vi "create_grid_from_corner_start.vi"(4 "y_step":dbl=0.1 format="%#_13g", 6 "x_step":dbl=0.1 format="%#_13g", 8 "y_n_pts":dbl=5.0 format="%#_13g", 9 "x_n_pts":dbl=5.0 format="%#_13g", 10 "y_start":dbl format="%#_13g", 11 "x_start":dbl format="%#_13g") -> (2 "Y":dbl[](array[numeric]), 3 "X":dbl[](array[numeric]))   [LabVIEW 2024]
uses:
  <vilib>/gmath/interp.llb/Create Mesh Grid (2D) (x,y arrays).vi
  <vilib>/gmath/NI_Gmath.lvlib
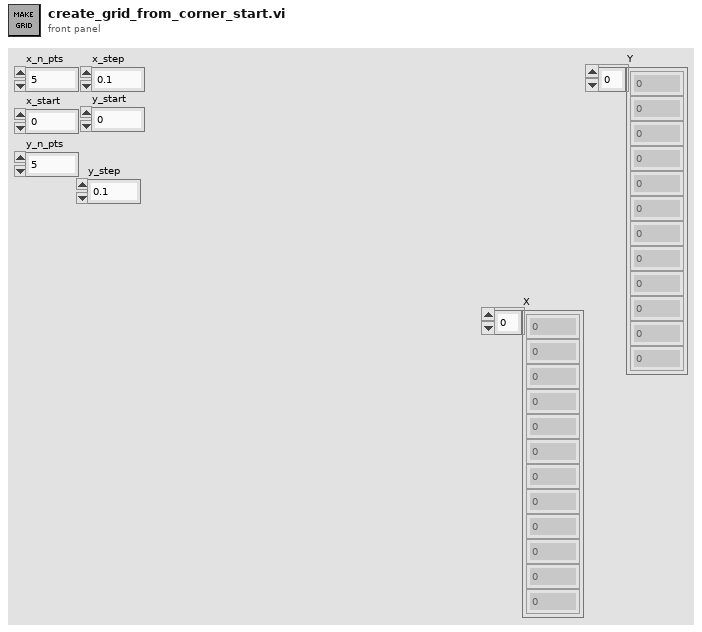
[diagram p1: front panel]
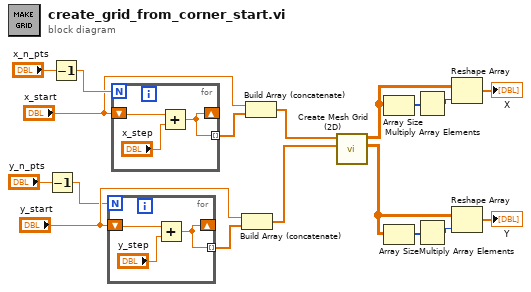
[diagram p0: block diagram]
diagram:
  n1 = Decrement(x="y_n_pts") -> (x-1=w12:dbl)
  n2 = Decrement(x="x_n_pts") -> (x-1=w17:dbl)
  n3 = for {
    N: w12 -> [_]
    shift-right: [w20] -> _
    shift-left: "y_start" -> [w21]
    tunnel: [w20] -> w13 mode=indexing
    n4 = Add(x=w21, y="y_step") -> (x+y=w20:dbl)
  }
  n5 = for {
    N: w17 -> [_]
    shift-right: [w23] -> _
    shift-left: "x_start" -> [w24]
    tunnel: [w23] -> w16 mode=indexing
    n6 = Add(x=w24, y="x_step") -> (x+y=w23:dbl)
  }
  n7 = Build Array (concatenate)("y_start", w13) -> (w9:dbl[])
  n8 = Build Array (concatenate)("x_start", w16) -> (w10:dbl[])
  n9 = call-poly <vilib>:"Create Mesh Grid (2D).vi"("y domain"=w9, "x domain"=w10) -> ("Y"=w1:dbl[][], "X"=w7:dbl[][])  [unwired: 7 in, 1 out]
  n10 = Array Size(array=w7) -> (size(s)=w6:i32[])
  n11 = Array Size(array=w1) -> (size(s)=w3:i32[])
  n12 = Multiply Array Elements(1:w6) -> (0:w5:i32)
  n13 = Multiply Array Elements(1:w3) -> (0:w4:i32)
  n14 = Reshape Array(w7, w5) -> (→"X":dbl[])
  n15 = Reshape Array(w1, w4) -> (→"Y":dbl[])
